vi "GiroL or GiroR.vi"() -> ()   [LabVIEW 2020]
panel:
  in  "GiroR":dbl
  in  "GiroL":dbl
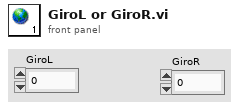
[diagram p1: front panel]
diagram:
